vi "SDO_SIM_SIM_Gyro_EXECUTE.vi"(6 "FPGA_Time_Seconds":dbl, 8 "error in (no error)":errorcluster) -> (0 "error out":errorcluster)   [LabVIEW 2019]
uses:
  Swerve_Drive_System/SDO_DRIVE_GLOBALS.vi
  SDO_SIM_SIM_Globals.vi
  <vilib>/Rock Robotics/WPI/ThirdParty/JAS_Junk/TrajLib/Trajectory_Library.lvlib
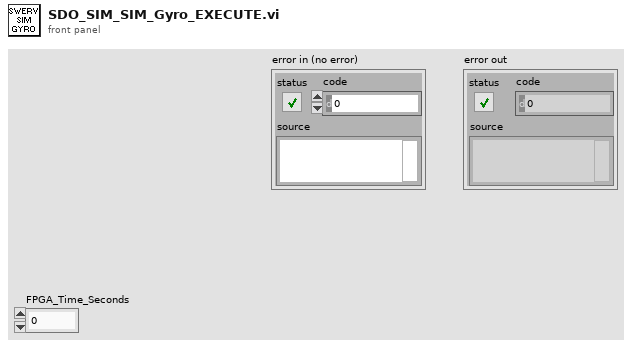
[diagram p1: front panel]
types:
  T1 = typedef "Trajectory_Library.lvlib/CHASSIS_SPEEDS.ctl" = cluster{"vX":dbl, "vY":dbl, "vOmega":dbl}
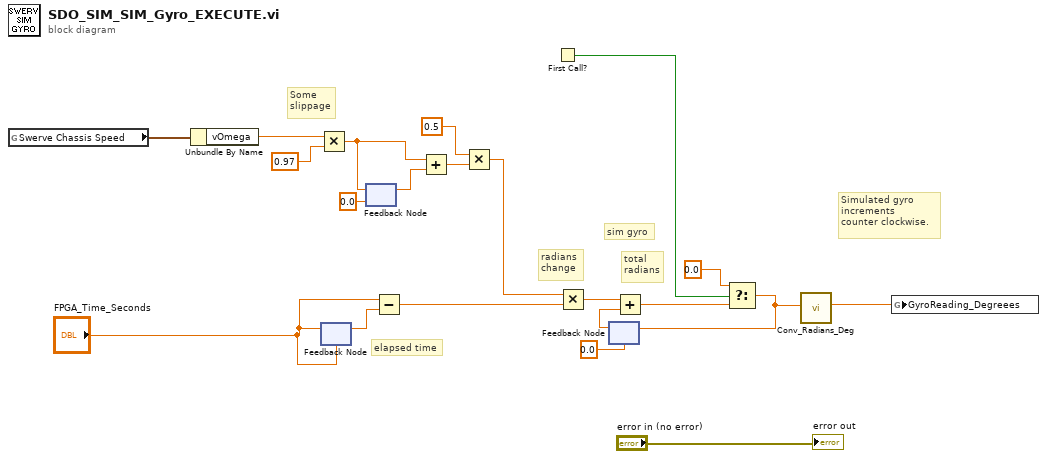
[diagram p0: block diagram]
diagram:
  # "Simulated gyro\nincrements\ncounter clockwise."
  # "Some \nslippage"
  # "elapsed time"
  # "total \nradians"
  # "radians \nchange"
  # "sim gyro"
  n1 = global read "SDO_DRIVE_GLOBALS.vi" "Swerve Chassis Speed"() -> (w21:T1)
  n2 = Unbundle By Name(w21) -> ("vOmega"=w20:dbl)
  n3 = Multiply(x=w20, y=0.97) -> (x*y=w6:dbl)
  n4 = feedback #1("FPGA_Time_Seconds") -> (w16:dbl)
  n5 = feedback-in #1("FPGA_Time_Seconds") -> ()
  n6 = feedback-in #2(w6) -> ()
  n7 = feedback #2(0.0) -> (w5:dbl)
  n8 = Subtract(x="FPGA_Time_Seconds", y=w16) -> (x-y=w15:dbl)
  n9 = Add(x=w6, y=w5) -> (x+y=w3:dbl)
  n10 = Multiply(x=0.5, y=w3) -> (x*y=w1:dbl)
  n11 = First Call?() -> (First Call?: T/F=w8:bool)
  n12 = Multiply(x=w1, y=w15) -> (x*y=w17:dbl)
  n13 = feedback #3(0.0) -> (w18:dbl)
  n14 = Add(x=w17, y=w18) -> (x+y=w10:dbl)
  n15 = Select(t=0.0, s=w8, f=w10) -> (s? t:f=w9:dbl)
  n16 = feedback-in #3(w9) -> ()
  n17 = call <vilib>:"Conv_Radians_Deg.vi"("Radians"=w9) -> ("Degrees"=w13:dbl)  [unwired: 10 in]
  n18 = global write "SDO_SIM_SIM_Globals.vi" "GyroReading_Degreees"(w13) -> ()
  "error out" <- "error in (no error)"
